vi "PKG_IMC_HandWheel1.vi"(9 "axis":i32, 10 "rate":dbl, 11 "Handle":u32) -> (2 "function return":i32, 3 "Handle out":u32)   [LabVIEW 2011, in "IMC_Pkg4xxx.lvlib"]
doc: "PKG_IMC_HandWheel1(IMC_HANDLE Handle, double rate, int axis);"
uses:
  IMC_Pkg4xxx.lvlib
  IMC_Pkg4xxx.dll
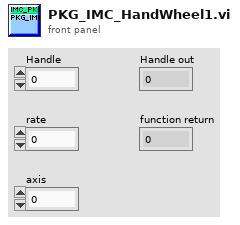
[diagram p1: front panel]
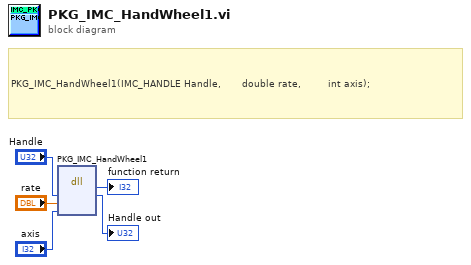
[diagram p0: block diagram]
diagram:
  # "PKG_IMC_HandWheel1(IMC_HANDLE Handle, \t\t\t\t\t\tdouble rate, \t\t\t\t\t\t\t\tint axis);"
  n1 = dll-call lib="PTH1mabs F光盘刻录\niMC MotionIMCNet_V4.0IMCAppincLabviewIMC_PKG4xxxIMC_PKG4xxx\nIMC_Pkg4xxx.*" fn="PKG_IMC_HandWheel1"("Handle"="Handle", "rate"="rate", "axis"="axis") -> (→"function return":i32, "Handle"=→"Handle out":u32)  [unwired: 5 in, 2 out]
